vi "Drag Edge Label.vi"(0 "FSM.Graph In":refnum<class "FSM.Graph.lvclass">, 9 "delta":T1) -> (4 "FSM.Graph Out":refnum<class "FSM.Graph.lvclass">)   [LabVIEW 2020, in "FSM.Graph.lvclass"]
uses:
  FSM.Graph.lvclass
  <vilib>/Utility/miscctls.llb/LVPoint32TypeDef.ctl
  FSM.Graph.lvclass/FSM.Graph.ctl
  FSM.Edge/FSM.Edge.lvclass
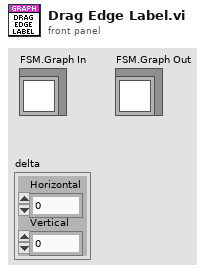
[diagram p1: front panel]
types:
  T1 = typedef "LVPoint32TypeDef.ctl" = cluster{"Horizontal":i32, "Vertical":i32}
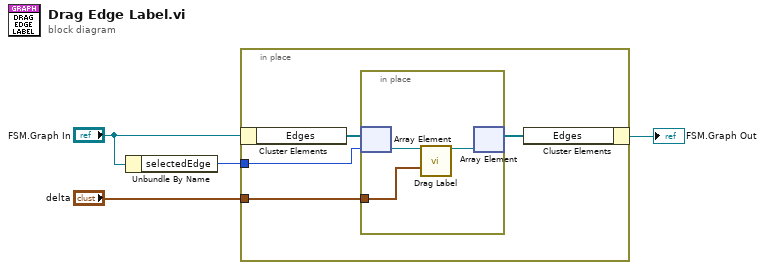
[diagram p0: block diagram]
diagram:
  n1 = Unbundle By Name("FSM.Graph In") -> ("selectedEdge"=w4:i32)
  n2 = in-place {
    in-place-border: w4 -> [w8]
    in-place-border: "delta" -> [w5]
    n3 = in-place-cluster #1("FSM.Graph In") -> ("Edges"=w7:refnum<class "FSM.Edge.lvclass">[])
    n4 = in-place {
      in-place-border: w5 -> [w9]
      n5 = in-place-array #2(w7, w8) -> (w11:refnum<class "FSM.Edge.lvclass">)
      n6 = call "Drag Label.vi"("FSM.Edge In"=w11, "delta"=w9) -> ("FSM.Edge Out"=w10:refnum<class "FSM.Edge.lvclass">)  [unwired: 13 in]
      n7 = in-place-array #2(w10) -> (w6:refnum<class "FSM.Edge.lvclass">[])  [unwired: 1 out]
    }
    n8 = in-place-cluster #1("Edges"=w6) -> (→"FSM.Graph Out":refnum<class "FSM.Graph.lvclass">)
  }
